vi "ATF-Storage-AO cluster to data.vi"(11 "output cluster":T1) -> (1 "Numeric":dbl, 2 "Component ID":string, 3 "Value":dbl, 5 "concatenated string":string)   [LabVIEW 2022 SP3]
doc: "This is an exclusive vi created to get the cluster data to Boolean ,String and Numeric"
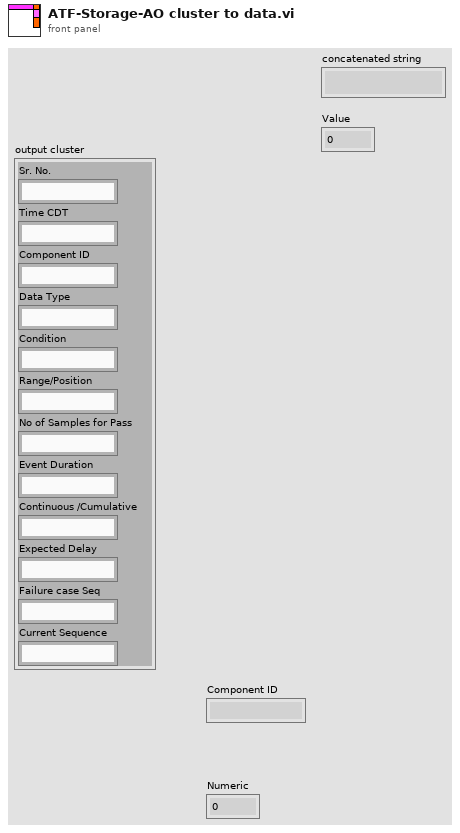
[diagram p1: front panel]
types:
  T1 = cluster{"Sr. No.":string, "Time CDT":string, "Component ID":string, "Data Type":string, "Condition":string, "Range/Position":string, "No of Samples for Pass":string, "Event Duration":string, "Continuous /Cumulative":string, "Expected Delay":string, "Failure case Seq":string, "Current Sequence":string}
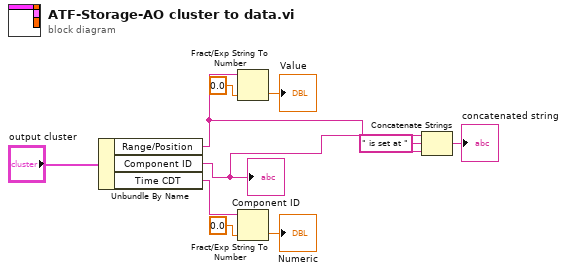
[diagram p0: block diagram]
diagram:
  n1 = Unbundle By Name("output cluster") -> ("Range/Position"=w4:string, "Component ID"=w3:string, "Time CDT"=w7:string)
  "Component ID" <- w3
  n2 = Fract/Exp String To Number(string=w4, default (0 dbl)=0.0 ("CDT")) -> (number=→"Value":dbl)  [unwired: 2 in, 1 out]
  n3 = Fract/Exp String To Number(string=w7, default (0 dbl)=0.0 ("CDT")) -> (number=→"Numeric":dbl)  [unwired: 2 in, 1 out]
  n4 = Concatenate Strings(w3, " is set at " ("string"), w4) -> (→"concatenated string":string)
